vi "basic_waveform_gen_dis.vi"() -> ()   [LabVIEW 2017]
panel:
  out "Waveform Graph":dbl[](graph)
  out "String":string
  in  "Upper Limit":dbl
  in  "Lower Limit":dbl
  out "Thermometer":dbl(slide) scale=0.0..100.0
  in  "stop":bool
  out "Waveform Chart":dbl(graph)
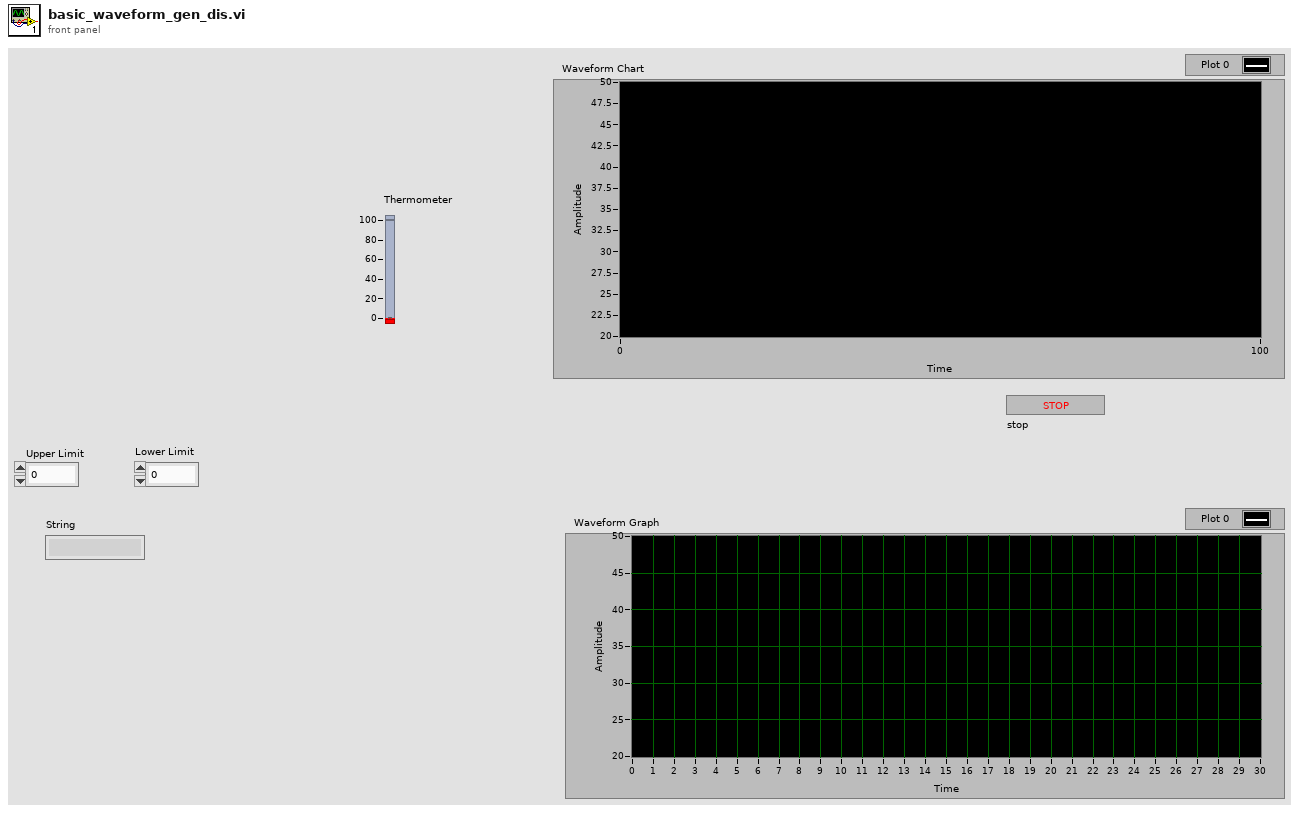
[diagram p1: front panel]
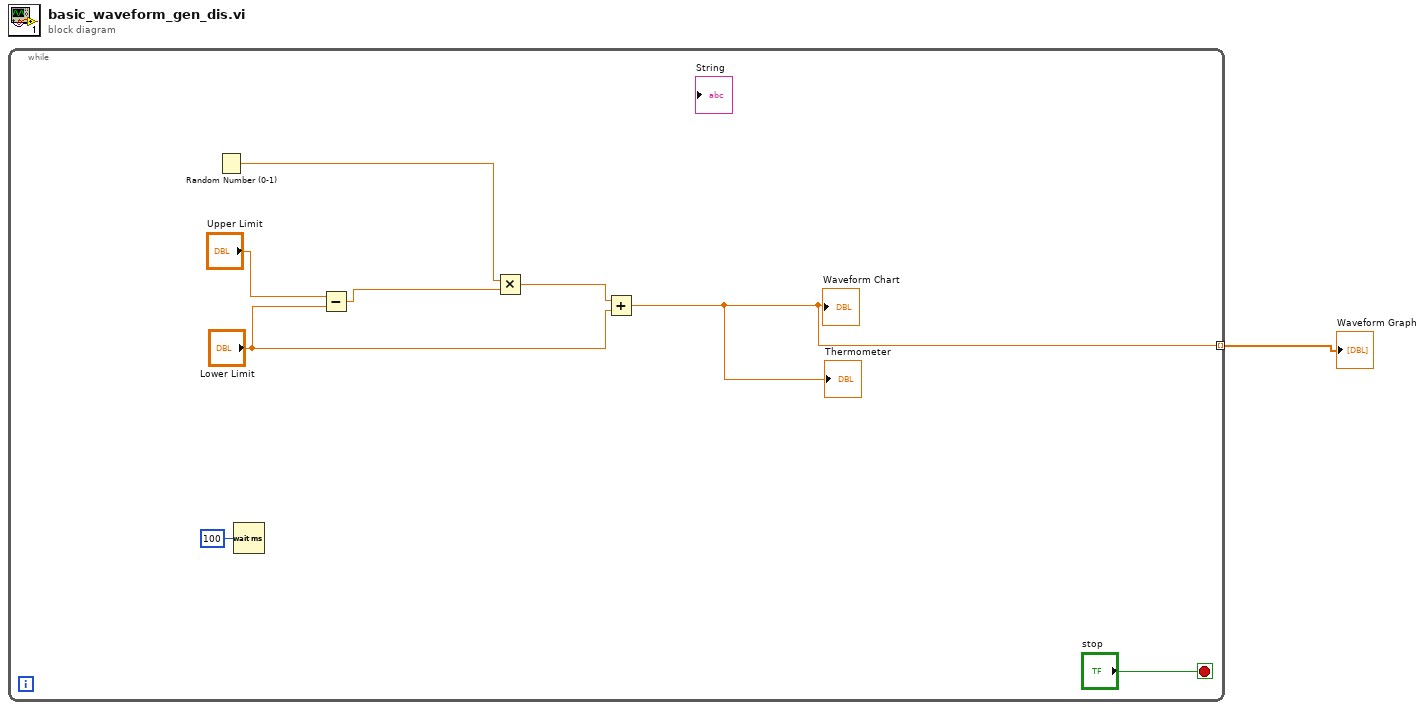
[diagram p0: block diagram]
diagram:
  n1 = while {
    tunnel: [w2] -> w1 mode=indexing
    stop <- "stop" stop-if-true
    n2 = Random Number (0-1)() -> (number: 0 to 1=w7:dbl)
    n3 = Wait (ms)(milliseconds to wait=u32 100) -> ()  [unwired: 1 out]
    n4 = Subtract(x="Upper Limit", y="Lower Limit") -> (x-y=w8:dbl)
    n5 = Multiply(x=w7, y=w8) -> (x*y=w6:dbl)
    n6 = Add(x=w6, y="Lower Limit") -> (x+y=w2:dbl)
    "Waveform Chart" <- w2
    "Thermometer" <- w2
  }
  "Waveform Graph" <- w1
